vi "UDP_robot.vi"   [LabVIEW 2011]
uses:
  signals/Signal.ctl
types:
  T1 = enum16{"Get Latest Data", "Get Local Data", "Get Remote Data", "Set Local Data", "Set Remote Data"}
  T2 = typedef "Signal.ctl" = enum16{"SIGFIRE", "SIGSTOPSCRIPT", "SIGSTARTGUN", "SIGSTOPGUN", "SIGDISABLED", "SIGENABLED", "SIGUDPTIMEOUT", "SIGNEWVISION_REMOTE", "SIGNEWVISION_LOCAL", "SIGSHOTFIRED", "SIGDOTRACK", "SIGDONTTRACK"}
  T3 = typedef "dashboard_return_data.ctl" = cluster{"Targetting Output":cluster{"X Position":dbl, "Distance":dbl, "Camera State":T4}, "Camera Error Status":errorcluster, "packet send timestamp":u32, "img process timestamp":u32}
  T4 = typedef "Camera State.ctl" = enum16{"No Targets", "Low Confidence", "Medium Confidence", "High Confidence", "Camera Error"}
  T5 = cluster{"X Position":dbl, "Distance":dbl, "Camera State":T4}
  T6 = typedef "WPI_CameraImageSize.ctl" = enum16{"640x480", "320x240", "160x120"}
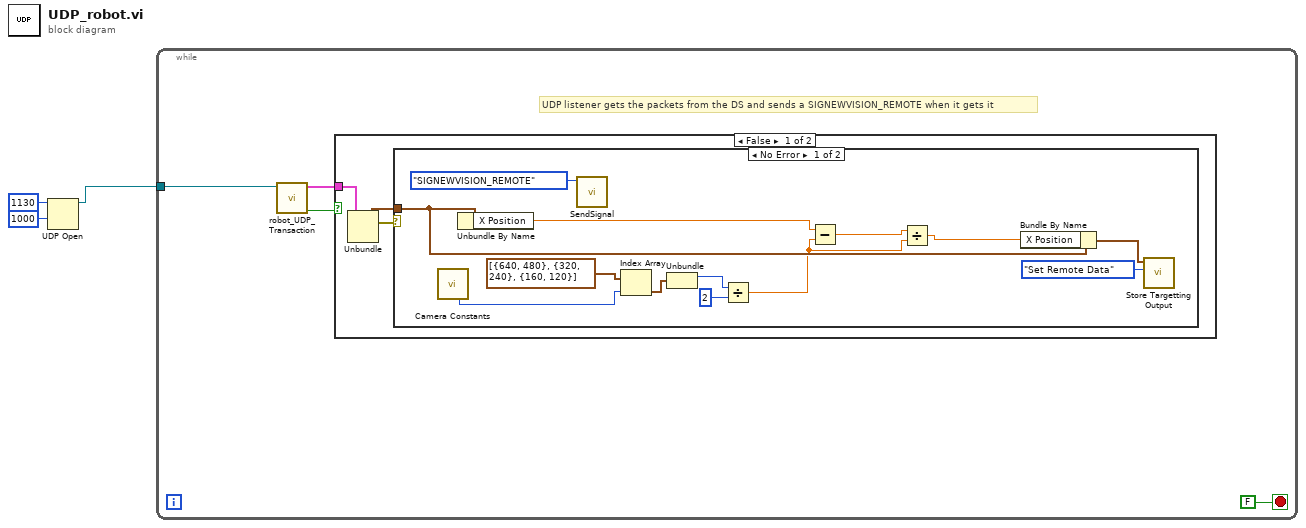
[diagram p0: block diagram]
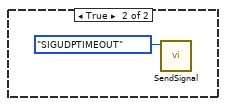
[diagram p3: hidden frame]
diagram:
  n1 = UDP Open(9:1000 ("timeout ms (25000)"), 11:u16 1130 ("port")) -> (port=w1:refnum<k16>)  [unwired: 3 in, 2 out]
  n2 = while {
    tunnel: w1 -> [w7]
    stop <- FALSE stop-if-true
    # "UDP listener gets the packets from the DS and sends a SIGNEWVISION_REMOTE when it gets it"
    n3 = call "robot_UDP_Transaction.vi"("connection ID"=w7) -> ("status"=w6:bool, "Dashboard Return Data"=w5:T3)  [unwired: 9 in]
    n4 = case shown="False" w6 {
      tunnel: w5 -> [w10 _]
      frame False {
        n5 = Unbundle(w10) -> ("Targetting Output"=w9:T5, "Camera Error Status"=w8:errorcluster)  [unwired: 2 out]
        n6 = case shown="No Error" w8 {
          tunnel: w9 -> [w21 _]
          frame No Error {
            n7 = call "Camera Constants.vi"() -> ("img size dashboard"=w18:T6)  [unwired: 5 in, 10 out]
            n8 = Unbundle By Name(w21) -> ("X Position"=w14:dbl)
            n9 = call "SendSignal.vi"("Signal"=Signal."SIGNEWVISION_REMOTE") -> ()  [unwired: 11 in]
            n10 = Index Array(array=cluster{i32, i32}[] [{640, 480}, {320, 240}, {160, 120}], index=w18) -> (element=w17:cluster{i32, i32})
            n11 = Unbundle(w17) -> (w16:i32)  [unwired: 1 out]
            n12 = Divide(x=w16, y=2) -> (x/y=w11:dbl)
            n13 = Subtract(x=w14, y=w11) -> (x-y=w13:dbl)
            n14 = Divide(x=w13, y=w11) -> (x/y=w12:dbl)
            n15 = Bundle By Name(cluster=w21, "X Position"=w12) -> (w20:T5)
            n16 = call "Store Targetting Output.vi"("mode"=T1."Set Remote Data", "Targetting Input"=w20) -> ()  [unwired: 9 in, 1 out]
          }
          frame Error {
          }
        }
      }
      frame True {
        n17 = call "SendSignal.vi"("Signal"=Signal."SIGUDPTIMEOUT") -> ()  [unwired: 11 in]
      }
    }
  }
